vi "Method_Const.vi"(4 "Value":cdb, 5 "Input A":T1) -> (1 "Result":T1)   [LabVIEW 2021, in "Divide_CPLX_DBL.lvclass"]
uses:
  Divide_CPLX_DBL.lvclass
  Abs Type.ctl
  Abs_Types/Complex Double Float/Abs_Complex Double Float.lvclass
  C:/Program Files (x86)/National Instruments/LabVIEW 2021/vi.lib/TSA/Abstract Data Classes/Abs_Types/Numeric/Abs_Numeric.lvclass
  C:/TSA/LV_Abstract/Source/Functions/Support/Function/Two Terminal/Cmplx DBL/AbsFunc_Two Term_Complex DBL.lvclass
  C:/Program Files (x86)/National Instruments/LabVIEW 2021/vi.lib/TSA/Abstract Data Classes/Abs_Types/Complex Double Float/Abs_Complex Double Float.lvclass
  Support/Function/Two Terminal/Cmplx DBL/AbsFunc_Two Term_Complex DBL.lvclass/AbsFunc_Two Term_Complex DBL.ctl
  Support/Function/Two Terminal/Cmplx DBL/Properties/Write Numeric A.vi
  Support/Function/Two Terminal/Cmplx DBL/Properties/Write Numeric B.vi
  Constants/Support/CPLX_DBL/Const_CPLX_DBL.lvclass
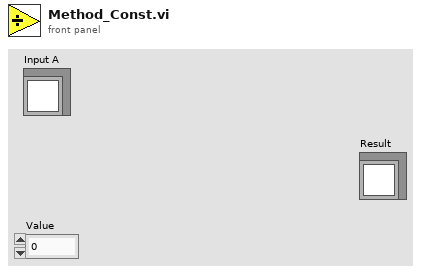
[diagram p1: front panel]
types:
  T1 = typedef "Divide_CPLX_DBL.lvclass/Abs Type.ctl" = refnum<class "Abs_Complex Double Float.lvclass">
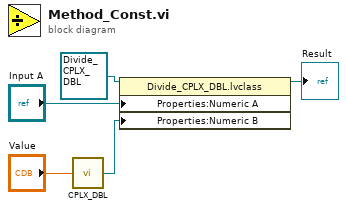
[diagram p0: block diagram]
diagram:
  n1 = call "CPLX_DBL.vi"("Value"="Value") -> ("Constant"=w2:refnum<class "Abs_Complex Double Float.lvclass">)  [unwired: 4 in]
  n2 = property class="Divide_CPLX_DBL.lvclass"(reference=refnum<class "Divide_CPLX_DBL.lvclass"> refnum ("Functions.lvlib:Numeric.lvlib:Divide.lvclass"), "Properties:Numeric A"="Input A", "Properties:Numeric B"=w2) -> (reference out=→"Result":refnum<class "Divide_CPLX_DBL.lvclass">)  [unwired: 1 in, 1 out]
